vi "count_reset.vi"(9 "reset":bool, 10 "inc":bool) -> (2 "sum 2":u8)   [LabVIEW 2018]
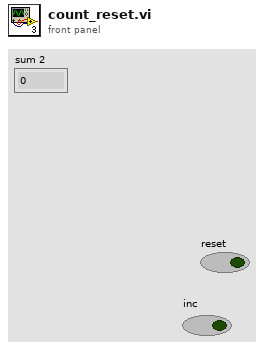
[diagram p1: front panel]
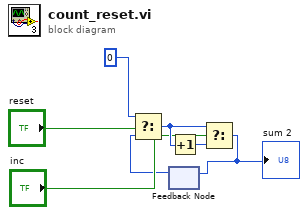
[diagram p0: block diagram]
diagram:
  n1 = feedback #1() -> (w1:u8)  [unwired: 1 in]
  n2 = Select(t=u8 0, s="reset", f=w1) -> (s? t:f=w4:u8)
  n3 = Increment(x=w4) -> (x+1=w5:u8)
  n4 = Select(t=w4, s="inc", f=w5) -> (s? t:f=w2:u8)
  "sum 2" <- w2
  n5 = feedback-in #1(w2) -> ()
